vi "Is Heart.vi"(7 "SS Image Path":path=path "C:/PokerSS/ViewSonic SS2.png", 8 "error in":errorcluster, 11 "ROI Descriptor (Heart Match)":T1={"Global Rectangle"=[530, 711, 555, 739], "Contours"=[{"ID"=enum."External", "Type"=12, "Coordinates"=[530, 711, 555, 739, 0]}]} {"Contours"."Type" items=["No Selection", "Point", "Line", "Rectangle", "Oval", "Polygon", "Freehand Region", "Annulus", "Unused2", "Unused3", "Broken Line", "Freehand Line", "Rotated Rectangle"]}) -> (0 "error out":errorcluster, 2 "Card Status":string, 3 "Found Heart":bool)   [LabVIEW 2015]
uses:
  <vilib>/vision/NI_Vision_Development_Module.lvlib
panel:
  in  "Template File Path (Heart Match)":path=path "C:/Users/Bob Dabalina/Documents/Labview/Poker Hand2/Heart Template.png"
  out "Image Out":T2(plugin-control)
  out "Matches (Heart Match)":T3(array[cluster]) {"Bounding Box"."y" format="%.2f"; "Bounding Box"."x" format="%.2f"; "Position"."y" format="%.2f"; "Position"."x" format="%.2f"; "Score" format="%.2f"; "Scale" format="%.2f"; "Angle" format="%.2f"}
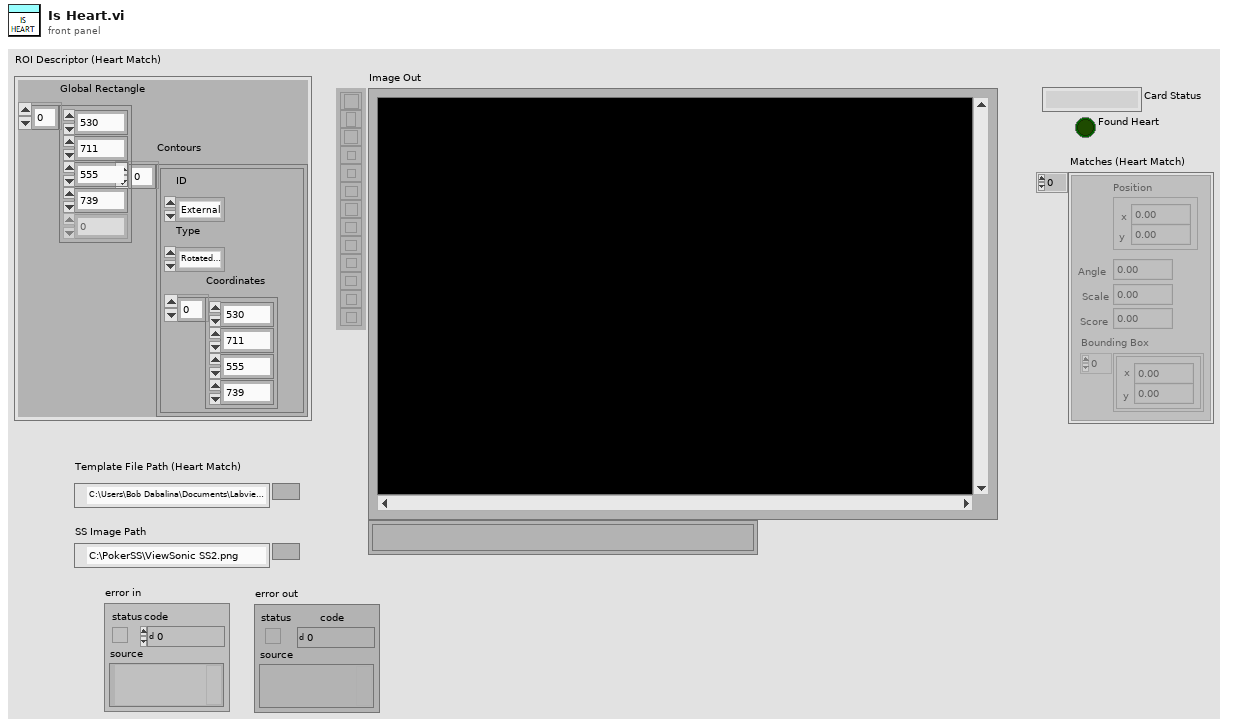
[diagram p1: front panel]
types:
  T1 = cluster{"Global Rectangle":i32[], "Contours":cluster{"ID":enum32{"External", "Internal"}, "Type":u32, "Coordinates":i32[]}[]}
  T2 = typedef "IMAQ Image.ctl" = refnum<image>
  T3 = cluster{"Position":cluster{"x":sgl, "y":sgl}, "Angle":sgl, "Scale":sgl, "Score":sgl, "Bounding Box":cluster{"x":sgl, "y":sgl}[]}[]
  T4 = cluster{"Number of Matches Requested":i32, "Minimum Match Score":sgl, "Angle Ranges":cluster{"Start Angle":sgl, "End Angle":sgl}[]}
  T5 = typedef "Image Type" = u32
  T6 = cluster{"Position":cluster{"x":sgl, "y":sgl}, "Angle":sgl, "Scale":sgl, "Score":sgl, "Bounding Box":cluster{"x":sgl, "y":sgl}[]}
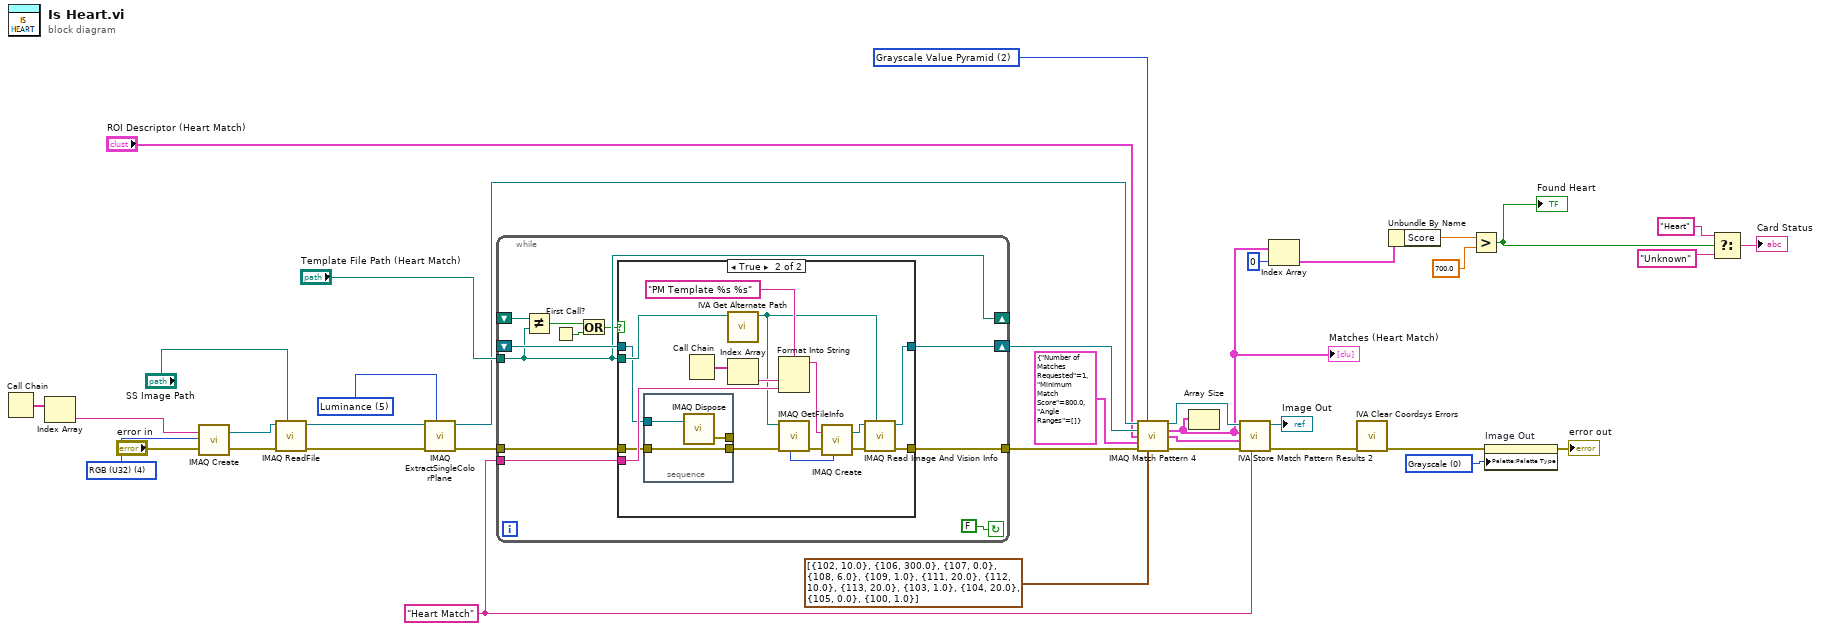
[diagram p0: block diagram]
diagram:
  w12 = u32 0 items=["Grayscale", "Binary", "Gradient", "Rainbow", "Temperature", "User Defined", "Binary 16 Bit", "Gradient 16 Bit", "Rainbow 16 Bit", "Temperature 16 Bit", "User Defined 16 Bit"] ("Palette Type")
  w23 = 2 items=["All", "Low Discrepancy Sampling", "Grayscale Value Pyramid", "Gradients Pyramid"] ("Algorithm")
  w21 = "Heart Match" ("Step Name")
  w30 = 5 items=["Red", "Green", "Blue", "Hue", "Saturation", "Luminance", "Value", "Intensity"] ("Color Plane")
  w31 = T5 4 items=["Grayscale (U8)", "Grayscale (I16)", "Grayscale (SGL)", "Complex (CSG)", "RGB (U32)", "HSL (U32)", "RGB (U64)", "Grayscale (U16)"] ("Image Type")
  n1 = Call Chain() -> (call chain=w33:string[])
  n2 = Index Array(array=w33) -> (element=w32:string)  [unwired: 1 in]
  n3 = call "IMAQ Create"("Image Name"=w32, "Image Type"=w31, "error in (no error)"="error in") -> ("New Image"=w36:T2, "error out"=w35:errorcluster)  [unwired: 1 in, 1 out]
  n4 = call "IMAQ ReadFile"("File Path"="SS Image Path", "error in (no error)"=w35, "Image"=w36) -> ("error out"=w37:errorcluster, "Image Out"=w29:T2)  [unwired: 2 in, 5 out]
  n5 = call "IMAQ ExtractSingleColorPlane"("Color Plane"=w30, "error in (no error)"=w37, "Image Src"=w29) -> ("error out"=w28:errorcluster, "Image Dst Out"=w26:T2)  [unwired: 1 in, 6 out]
  n6 = while {
    shift-right: [w48] -> w19
    shift-left: _ -> [w47]
    tunnel: [w45] -> w18
    tunnel: w28 -> [w44]
    tunnel: "Template File Path (Heart Match)" -> [w41]
    tunnel: w21 -> [w43]
    shift-right: [w41] -> _
    shift-left: _ -> [w42]
    stop <- FALSE continue-if-true
    n7 = Not Equal?(x=w42, y=w41) -> (x != y?=w39:bool)
    n8 = First Call?() -> (First Call?: T/F=w40:bool)
    n9 = Or(x=w39, y=w40) -> (x .or. y?=w38:bool)
    n10 = case shown="True" w38 {
      tunnel: [w50 w64] -> w48
      tunnel: w47 -> [w50 w56]
      tunnel: [w49 w61] -> w45
      tunnel: w44 -> [w49 w55]
      tunnel: w41 -> [_ w57]
      tunnel: w43 -> [_ w58]
      frame False {
      }
      frame True {
        n11 = stacked-sequence {
          tunnel: w56 -> [w69]
          tunnel: w55 -> [w68]
          tunnel: [w68] -> w51
          tunnel: [w67] -> _
          frame #0 {
            n12 = call "IMAQ Dispose"("Image"=w69) -> ("error out"=w67:errorcluster)  [unwired: 2 in, 3 out]
          }
        }
        n13 = Call Chain() -> (call chain=w60:string[])
        n14 = call <vilib>:"IVA Get Alternate Path.vi"("Path In"=w57) -> ("Path Out"=w53:path)  [unwired: 10 out]
        n15 = Index Array(array=w60) -> (element=w59:string)  [unwired: 1 in]
        n16 = Format Into String(format string="PM Template %s %s" ("Image Name"), w59, w58) -> (resulting string=w66:string)  [unwired: 2 in, 1 out]
        n17 = call "IMAQ GetFileInfo"("error in (no error)"=w51, "File Path"=w53) -> ("error out"=w52:errorcluster, "Image Type"=w54:T5)  [unwired: 3 in, 5 out]
        n18 = call "IMAQ Create"("Image Name"=w66, "Image Type"=w54, "error in (no error)"=w52) -> ("New Image"=w63:T2, "error out"=w62:errorcluster)  [unwired: 1 in, 1 out]
        n19 = call "IMAQ Read Image And Vision Info"("File Path"=w53, "error in (no error)"=w62, "Image"=w63) -> ("error out"=w61:errorcluster, "Image Out"=w64:T2)  [unwired: 1 in, 6 out]
      }
    }
  }
  n20 = call "IMAQ Match Pattern 4"("Image"=w26, "Algorithm"=w23, "Template Image"=w19, "ROI Descriptor"="ROI Descriptor (Heart Match)", "Parameters"=T4 {"Number of Matches Requested"=1, "Minimum Match Score"=800.0, "Angle Ranges"=[]}, "error in (no error)"=w18, "Advanced Options"=cluster{"Item":u16, "Value":dbl}[] [{"Item"=102, "Value"=10.0}, {"Item"=106, "Value"=300.0}, {"Item"=107, "Value"=0.0}, {"Item"=108, "Value"=6.0}, {"Item"=109, "Value"=1.0}, {"Item"=111, "Value"=20.0}, {"Item"=112, "Value"=10.0}, {"Item"=113, "Value"=20.0}, {"Item"=103, "Value"=1.0}, {"Item"=104, "Value"=20.0}, {"Item"=105, "Value"=0.0}, {"Item"=100, "Value"=1.0}]) -> ("Image (duplicate)"=w24:T2, "Matches (pixel)"=w9:T3, "Matches (real-world)"=w20:T3, "error out"=w25:errorcluster)  [unwired: 4 in, 1 out]
  "Matches (Heart Match)" <- w9
  n21 = Array Size(array=w9) -> ()  [unwired: 1 out]
  n22 = call <vilib>:"IVA Store Match Pattern Results 2.vi"("Step Name"=w21, "error in (no error)"=w25, "Matches (real-world)"=w20, "Matches (pixel)"=w9, "Image in"=w24) -> ("error out"=w17:errorcluster, "Image dup"=→"Image Out":T2)  [unwired: 1 in, 4 out]
  n23 = Index Array(array=w9, index=0) -> (element=w8:T6)
  n24 = call <vilib>:"IVA Clear Coordsys Errors.vi"("error in (no error)"=w17) -> ("error out"=w16:errorcluster)  [unwired: 10 in]
  n25 = Unbundle By Name(w8) -> ("Score"=w7:sgl)
  n26 = Greater?(x=w7, y=sgl 700.0) -> (0:w1:bool)
  "Found Heart" <- w1
  n27 = property on="Image Out" class="ImageControl"(error in=w16, "Palette:Palette Type"=w12) -> (error out=→"error out":errorcluster)  [unwired: 1 in, 1 out]
  n28 = Select(t="Heart", s=w1, f="Unknown") -> (s? t:f=→"Card Status":string)
